vi "Get Strings.vi"(8 "error in (no error)":errorcluster, 11 "Buffer in":refnum<class "Unique String Buffer.lvclass">) -> (0 "error out":errorcluster, 2 "strings":string[](array[string]), 3 "Buffer out":refnum<class "Unique String Buffer.lvclass">)   [LabVIEW 2015, in "SLSC Switch.lvlib" / "Unique String Buffer.lvclass"]
uses:
  Unique String Buffer.lvclass
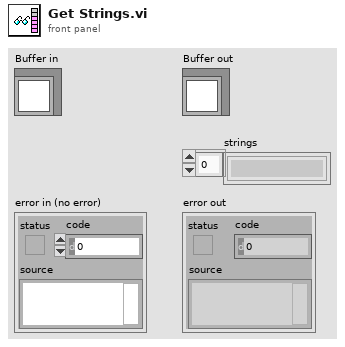
[diagram p1: front panel]
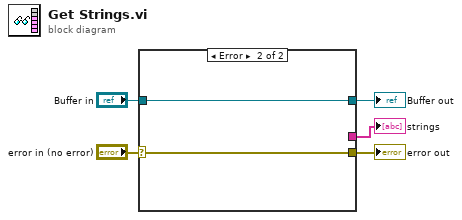
[diagram p0: block diagram]
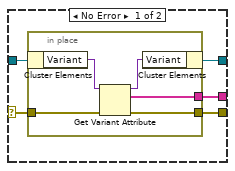
[diagram p2: hidden frame]
diagram:
  n1 = case shown="Error" "error in (no error)" {
    selector: "error in (no error)" -> [w7 w17]
    tunnel: [w6 w17] -> w4
    tunnel: [w9 w16] -> w2
    tunnel: "Buffer in" -> [w10 w16]
    tunnel: [w8 _] -> w1
    frame No Error {
      n2 = in-place {
        in-place-border: [w13] -> w8
        in-place-border: w7 -> [w12]
        in-place-border: [w11] -> w6
        n3 = in-place-cluster #1(w10) -> ("Variant"=w15:variant)
        n4 = Get Variant Attribute(Variant=w15, error in=w12) -> (duplicate Variant=w14:variant, names=w13:string[], error out=w11:errorcluster)  [unwired: 2 in, 1 out]
        n5 = in-place-cluster #1("Variant"=w14) -> (w9:refnum<class "Unique String Buffer.lvclass">)
      }
    }
    frame Error {
    }
  }
  "error out" <- w4
  "Buffer out" <- w2
  "strings" <- w1
